vi "Read DAC Settings.vi"(11 "ILC in":refnum<class "ILC.lvclass">) -> (2 "DAC Settings":T1={"Voltage Reference"=4.096, "Min Counts"=0, "Max Counts"=65535} {"Voltage Reference" format="%.3f"}, 3 "ILC out":refnum<class "ILC.lvclass">)   [LabVIEW 2015, in "ILCCommon.lvlib" / "ILC.lvclass"]
uses:
  <userlib>/Common/ILC/ILC/ILC.lvclass
  <userlib>/Common/ILC/Typedefs/DAC Settings.ctl
  <userlib>/Common/ILC/ILC/ILC.lvclass/ILC.ctl
  <userlib>/Common/ILC/Typedefs/ILCTypedefs.lvlib
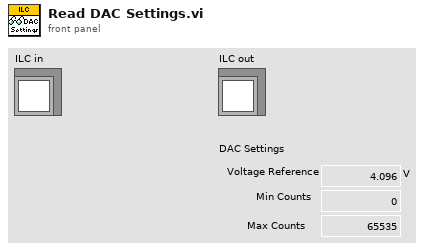
[diagram p1: front panel]
types:
  T1 = typedef "ILCCommon.lvlib/ILCTypedefs.lvlib/DAC Settings.ctl" = cluster{"Voltage Reference":dbl[unit], "Min Counts":i32, "Max Counts":i32}
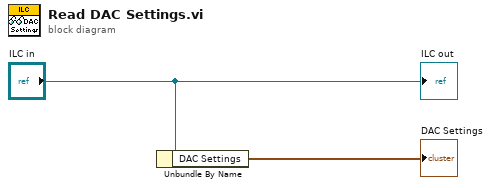
[diagram p0: block diagram]
diagram:
  n1 = Unbundle By Name("ILC in") -> ("DAC Settings"=→"DAC Settings":T1)
  "ILC out" <- "ILC in"
